vi "TagDB Refmgr-Defer Panel Update.vi"(8 "error in (no error)":errorcluster, 9 "Defer Updates?":bool, 10 "Key":string, 11 "TagDB in":T1) -> (0 "error out":errorcluster, 3 "TagDB out":T1)   [LabVIEW 2017, in "TagDB RefManager.lvlib"]
uses:
  TagDB RefManager.lvlib
  <userlib>/_NEVSTOP/TagDB/Typedef/TagDB.ctl
  2fcb9fa5-0483-4838-9848-5a7367d2b499.vi
  2fcb9fa5-0483-4838-9848-5a7367d2b499.vi/44092bd3-709c-4e20-87d5-ef7c9706681c.vi
  <userlib>/_NEVSTOP/TagDB/_Support/Change Detector/TagDB dbChanged.vi
  2fcb9fa5-0483-4838-9848-5a7367d2b499.vi/44092bd3-709c-4e20-87d5-ef7c9706681c.vi/29b2ea6d-6d7f-4e4a-ad31-a5cb760462c7.vi
  <userlib>/_NEVSTOP/TagDB/API/TagDB-Status.vi
  <userlib>/_NEVSTOP/TagDB/_Support/Change Detector/TagDB ChangeFlag.vi
  <userlib>/_NEVSTOP/TagDB/_Support/DataAccess/_NameCacher.vi
  <userlib>/_NEVSTOP/TagDB/_Support/DataAccess/TagDB Ref to DVR.vi
  <userlib>/_NEVSTOP/TagDB/_Support/URL/TRIM-BOTH-SPACE.vi
  <userlib>/_NEVSTOP/TagDB/_Support/Error/_[error50000]Invalid DB REF.vi
  <userlib>/_NEVSTOP/TagDB/_Support/Error/_[error50002]Invalid DataType.vi
  <userlib>/_NEVSTOP/TagDB/_Support/Error/_Clear Errors.vi
  _Support/Error/[-50011] Instance Not Found.vi
  _Support/Error/[-50010] Mutiple Instances.vi
  <userlib>/_NEVSTOP/TagDB/TagDB.lvlib
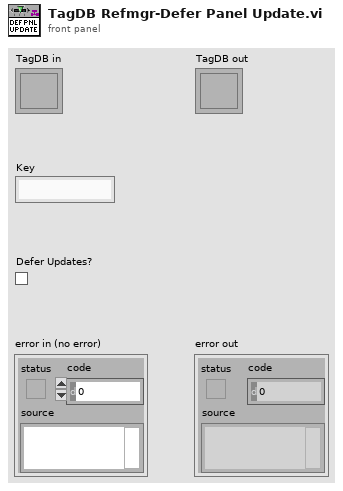
[diagram p1: front panel]
types:
  T1 = typedef "TagDB.lvlib/TagDB.ctl" = refnum<k1>
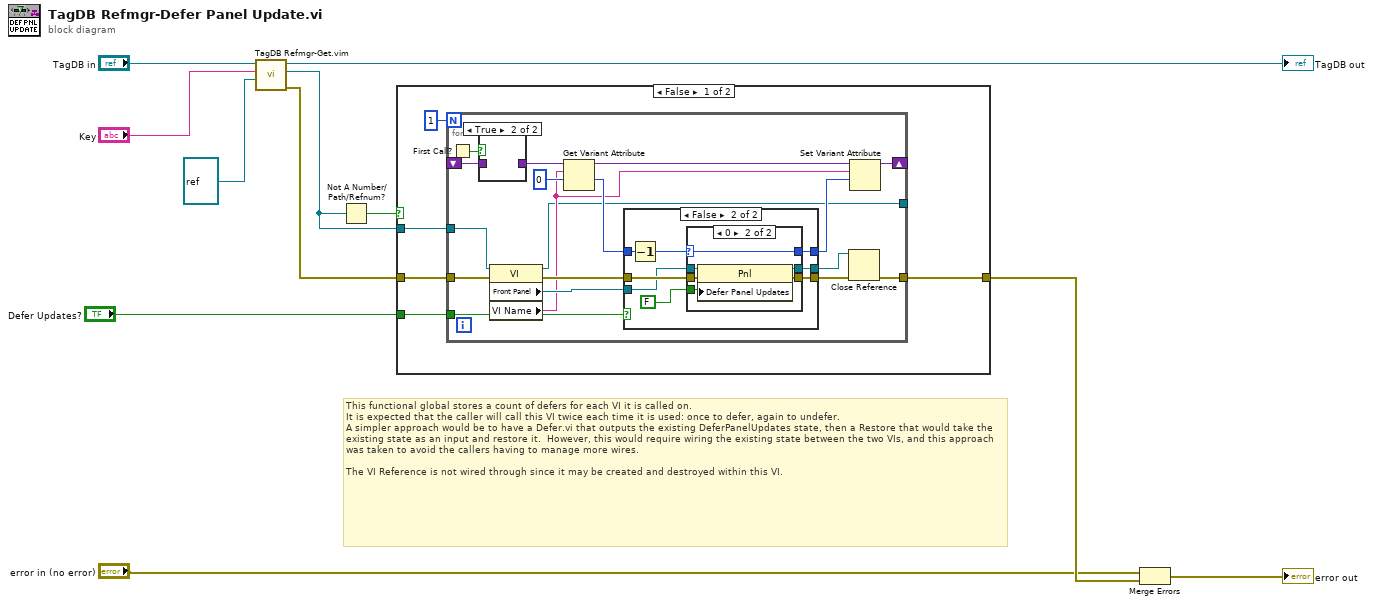
[diagram p0: block diagram]
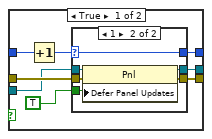
[diagram p3: hidden frame]
diagram:
  # "This functional global stores a count of defers for each VI it is called on.\nIt is expected that the caller will call this VI twice each time it is used: once to defer, again to undefer.\nA simpler approach would be to have a Defer.vi that outputs the existing DeferPanelUpdates state, then a Restore that would take the existing state as an input and restore it.  However, this would require wiring the existing state between the two VIs, and this approach was taken to avoid the callers having to manage more wires.\n\nThe VI Reference is not wired through since it may be created and destroyed within this VI."
  n1 = call "TagDB Refmgr-Get.vim"("Type"=refnum<vi> refnum ("VI Refnum"), "RegExp"="Key", "DB Ref"="TagDB in") -> ("error out"=w1:errorcluster, "Reference"=w6:refnum<vi>, "DB Ref(dup)"=→"TagDB out":T1)  [unwired: 5 in, 1 out]
  n2 = Not A Number/Path/Refnum?(number/path/refnum=w6) -> (NaN/Path/Refnum?=w2:bool)
  n3 = case shown="False" w2 {
    tunnel: "Defer Updates?" -> [w16 _]
    tunnel: w6 -> [w15 _]
    tunnel: [w13 _] -> w5
    tunnel: w1 -> [w12 _]
    frame False {
      n4 = for {
        N: 1 -> [_]
        shift-right: [w34] -> _
        shift-left: _ -> [w26]
        tunnel: w15 -> [w19]
        tunnel: w16 -> [w30]
        tunnel: [w18] -> _
        tunnel: [w20] -> w13
        tunnel: w12 -> [w17]
        n5 = First Call?() -> (First Call?: T/F=w27:bool)
        n6 = case shown="True" w27 {
          tunnel: w26 -> [w35 _]
          tunnel: [w35 _] -> w25
          frame False {
          }
          frame True {
          }
        }
        n7 = property class="VI"(reference=w19, error in=w17) -> (reference out=w18:refnum<vi>, error out=w31:errorcluster, "Front Panel"=w28:refnum<vi>, "VI Name"=w23:string)
        n8 = Get Variant Attribute(Variant=w25, name=w23, default value (empty Variant)=0) -> (duplicate Variant=w33:variant, value=w29:i32)  [unwired: 1 in, 2 out]
        n9 = case shown="False" w30 {
          tunnel: w31 -> [w43 w60]
          tunnel: w29 -> [w38 w55]
          tunnel: w28 -> [w42 w59]
          tunnel: [w41 w58] -> w22
          tunnel: [w36 w53] -> w24
          tunnel: [w39 w56] -> w21
          frame True {
            n10 = Increment(x=w38) -> (x+1=w37:i32)
            n11 = case shown="1" w37 {
              selector: w37 -> [w44 w47]
              tunnel: w43 -> [w46 w52]
              tunnel: w42 -> [w45 w51]
              tunnel: TRUE -> [_ w50]
              tunnel: [w46 w49] -> w41
              tunnel: [w45 w48] -> w39
              tunnel: [w44 w47] -> w36
              frame Default {
              }
              frame 1 {
                n12 = property class="Pnl"(reference=w51, error in=w52, "Defer Panel Updates"=w50) -> (reference out=w48:refnum<vi>, error out=w49:errorcluster)
              }
            }
          }
          frame False {
            n13 = Decrement(x=w55) -> (x-1=w54:i32)
            n14 = case shown="0" w54 {
              selector: w54 -> [w61 w64]
              tunnel: w60 -> [w63 w69]
              tunnel: w59 -> [w62 w68]
              tunnel: FALSE -> [_ w67]
              tunnel: [w63 w66] -> w58
              tunnel: [w62 w65] -> w56
              tunnel: [w61 w64] -> w53
              frame Default {
              }
              frame 0 {
                n15 = property class="Pnl"(reference=w68, error in=w69, "Defer Panel Updates"=w67) -> (reference out=w65:refnum<vi>, error out=w66:errorcluster)
              }
            }
          }
        }
        n16 = Close Reference(reference=w21, error in (no error)=w22) -> (error out=w20:errorcluster)
        n17 = Set Variant Attribute(Variant=w33, name=w23, value=w24) -> (Variant out=w34:variant)  [unwired: 1 in, 2 out]
      }
    }
    frame True {
    }
  }
  n18 = Merge Errors("error in (no error)", w5) -> (→"error out":errorcluster)
